vi "Teardown - Forrmat Variant Into String.vi"(8 "error in (no error)":errorcluster, 11 "Refnum":refnum<file>) -> (0 "error out":errorcluster)   [LabVIEW 2009]
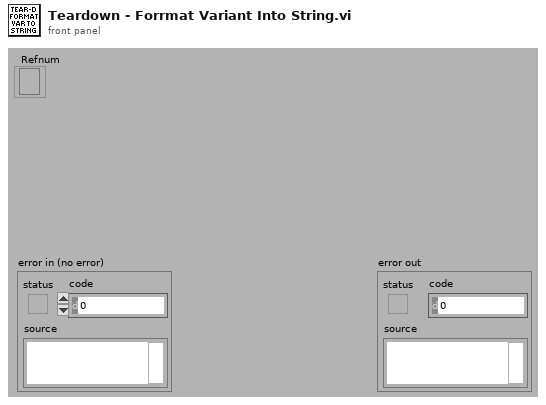
[diagram p1: front panel]
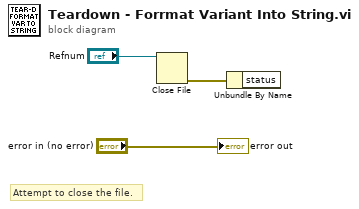
[diagram p0: block diagram]
diagram:
  # "Attempt to close the file."
  n1 = Close File(refnum="Refnum") -> (error out=w2:errorcluster)  [unwired: 1 in, 1 out]
  n2 = Unbundle By Name(w2) -> ()  [unwired: 1 out]
  "error out" <- "error in (no error)"
